vi "GetID.vi"(8 "error in (no error)":errorcluster, 11 "reference in":refnum<class "Rig.lvclass">) -> (0 "error out":errorcluster, 2 "Id String":string, 3 "reference in":refnum<class "Rig.lvclass">)   [LabVIEW 2020, in "Rig.lvclass"]
uses:
  Rig.lvclass
  Equipment_class/Equipment.lvclass
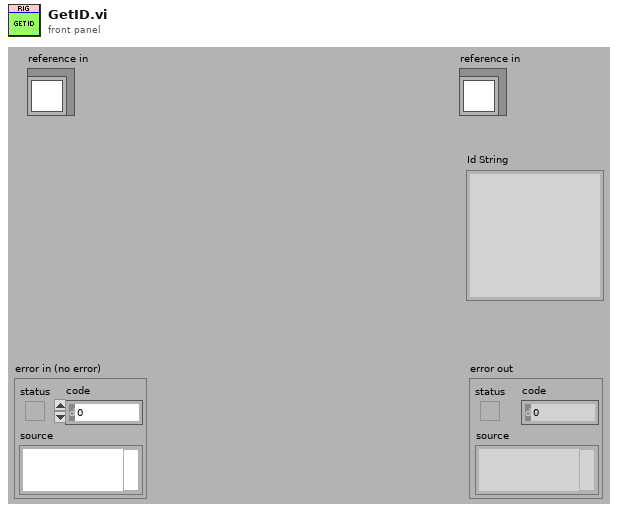
[diagram p1: front panel]
types:
  T1 = typedef "Rig.lvclass/ObjectAttributes.ctl" = cluster{"Children":refnum<class "Equipment.lvclass">[]}
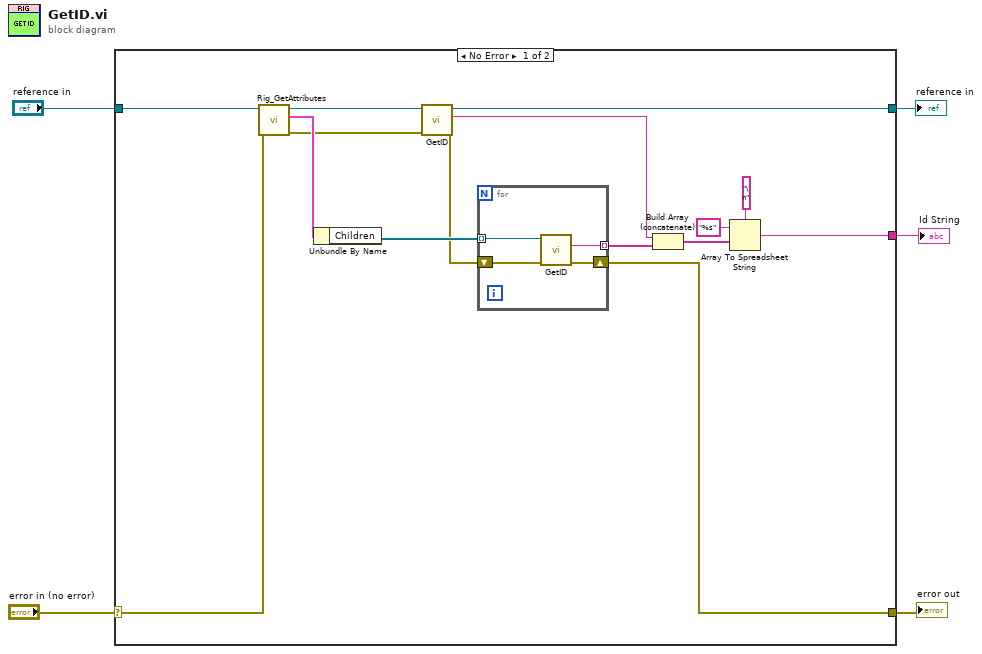
[diagram p0: block diagram]
diagram:
  n1 = case shown="No Error" "error in (no error)" {
    selector: "error in (no error)" -> [w20 w26]
    tunnel: [w12 w26] -> w4
    tunnel: [w16 w25] -> w2
    tunnel: "reference in" -> [w18 w25]
    tunnel: [w6 _] -> w1
    frame No Error {
      n2 = call "Rig_GetAttributes.vi"("error in (no error)"=w20, "reference in"=w18) -> ("error out"=w13:errorcluster, "Data"=w19:T1, "reference out"=w17:refnum<class "Rig.lvclass">)  [unwired: 6 in, 1 out]
      n3 = Unbundle By Name(w19) -> ("Children"=w15:refnum<class "Equipment.lvclass">[])
      n4 = call-parent "GetID.vi"("error in (no error)"=w13, "reference in"=w17) -> ("error out"=w14:errorcluster, "Id String"=w11:string, "reference out"=w16:refnum<class "Rig.lvclass">)  [unwired: 7 in]
      n5 = for {
        tunnel: w15 -> [w24] mode=indexing
        shift-right: [w22] -> w12
        shift-left: w14 -> [w23]
        tunnel: [w21] -> w10 mode=indexing
        n6 = call-dynamic "GetID.vi"("error in (no error)"=w23, "reference in"=w24) -> ("error out"=w22:errorcluster, "Id String"=w21:string)  [unwired: 7 in, 1 out]
      }
      n7 = Build Array (concatenate)(w11, w10) -> (w9:string[])
      n8 = Array To Spreadsheet String(delimiter (Tab)="\n", array=w9, 3:"%s" ("format string")) -> (spreadsheet string=w6:string)
    }
    frame Error {
    }
  }
  "error out" <- w4
  "reference in" <- w2
  "Id String" <- w1
